vi "matrix.vi"() -> ()   [LabVIEW 2018]
uses:
  <vilib>/Analysis/Matrix/Datatypes/RealMatrix.ctl
  c9e6c382-d998-434b-854e-66d4fe045495.vi
  328defa3-4063-475c-9f4d-f61dd8250632.vi
  <vilib>/Array/Sort 2D Array - Pop Stack.vi
  <vilib>/Array/Sort 2D Array - Push Stack.vi
  <vilib>/Analysis/Matrix/NI_Matrix.lvlib
panel:
  out "min index(es)":i32
  out "min value 2":dbl
  out "max index(es)":i32
  out "max value 2":dbl
  in  "array":dbl[](array[numeric])
  out "min value":dbl
  out "max value":dbl
  out "sorted 2D array 2":T1
  out "sorted 2D array":T1
  in  "rows":dbl
  out "appended array":T1
  in  "columns":dbl
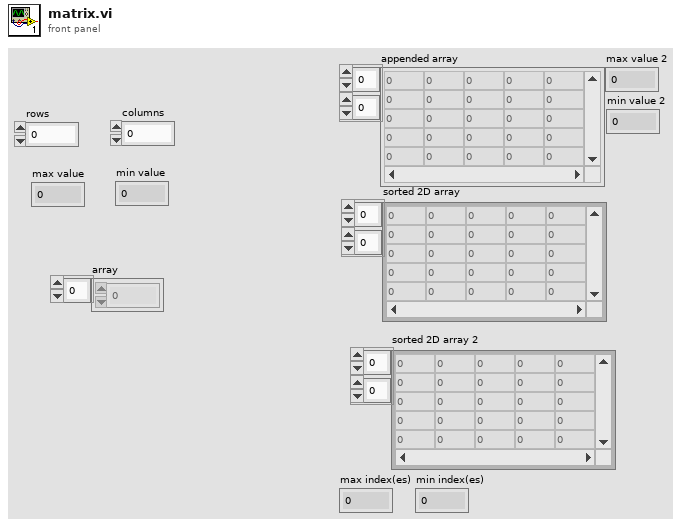
[diagram p1: front panel]
types:
  T1 = typedef "NI_Matrix.lvlib/RealMatrix.ctl" = dbl[][]
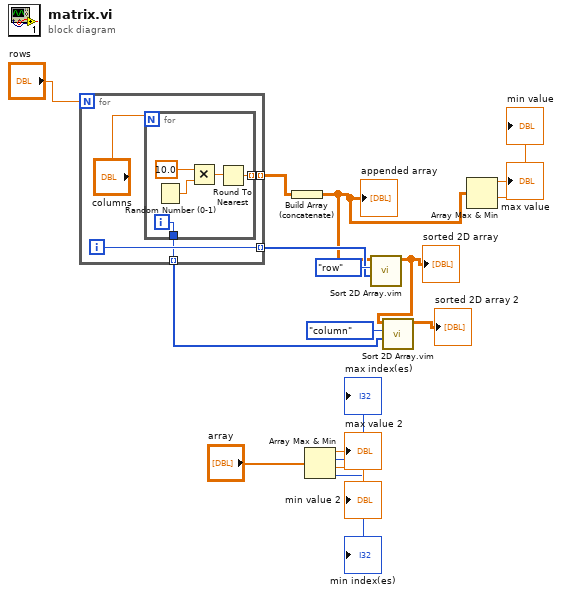
[diagram p0: block diagram]
diagram:
  n1 = for {
    N: "rows" -> [_]
    tunnel: [w19] -> w15 mode=indexing
    tunnel: [w18] -> w13 mode=indexing
    tunnel: [w17] -> w9 mode=indexing
    i -> [w18]
    n2 = for {
      N: "columns" -> [_]
      tunnel: [w22] -> w19 mode=indexing
      tunnel: [w21] -> w17
      i -> [w21]
      n3 = Random Number (0-1)() -> (number: 0 to 1=w25:dbl)
      n4 = Multiply(x=10.0, y=w25) -> (x*y=w23:dbl)
      n5 = Round To Nearest(number=w23) -> (nearest integer value=w22:dbl)
    }
  }
  n6 = Build Array (concatenate)(w15) -> (w8:T1)
  "appended array" <- w8
  n7 = Array Max & Min(array="array") -> (max value=→"max value 2":dbl, max index (indices)=→"max index(es)":i32, min value=→"min value 2":dbl, min index (indices)=→"min index(es)":i32)
  n8 = call "Sort 2D Array.vim"("index"=w13, "dimension to index (column)"=enum16{"column", "row"}."row", "2D array"=w8) -> ("sorted 2D array"=w11:T1)  [unwired: 7 in, 1 out]
  "sorted 2D array" <- w11
  n9 = call "Sort 2D Array.vim"("index"=w9, "dimension to index (column)"=enum16{"column", "row"}."column", "2D array"=w11) -> ("sorted 2D array"=→"sorted 2D array 2":T1)  [unwired: 7 in, 1 out]
  n10 = Array Max & Min(array=w8) -> (max value=→"max value":dbl, min value=→"min value":dbl)  [unwired: 2 out]
